vi "Caller VI_Read Icon Data From Tag.vi"(8 "Error":errorcluster, 11 "Default Body Text":T2 {"Body Text Spec"."Alignment" items=["left", "center", "right"]}) -> (0 "Error Out":errorcluster, 1 "Library Icon If Valid":picture, 2 "Who Invoked The Icon Editor? Out":T5, 3 "Data Out":T1 {"Body Text"."Body Text Spec"."Alignment" items=["left", "center", "right"]}, 4 "Valid? Out":bool, 5 "Valid Library Icon? Out":bool)   [LabVIEW 2021]
uses:
  <resource>/plugins/IconEditor/Who Invoked Icon Editor.ctl
  <resource>/plugins/IconEditor/Icon Editor Invoker Type.ctl
  TypeDefs/Cluster_BodyText.ctl
  vi.lib/LabVIEW Icon API/lv_icon/Controls/Font.ctl
  vi.lib/LabVIEW Icon API/lv_icon/Controls/Alignment.ctl
  vi.lib/LabVIEW Icon API/lv_icon/Controls/LabVIEW Icon Stored Information.ctl
  vi.lib/LabVIEW Icon API/lv_icon/Classes/Layer/Layer.lvclass
  vi.lib/LabVIEW Icon API/lv_icon/lv_icon.lvlib
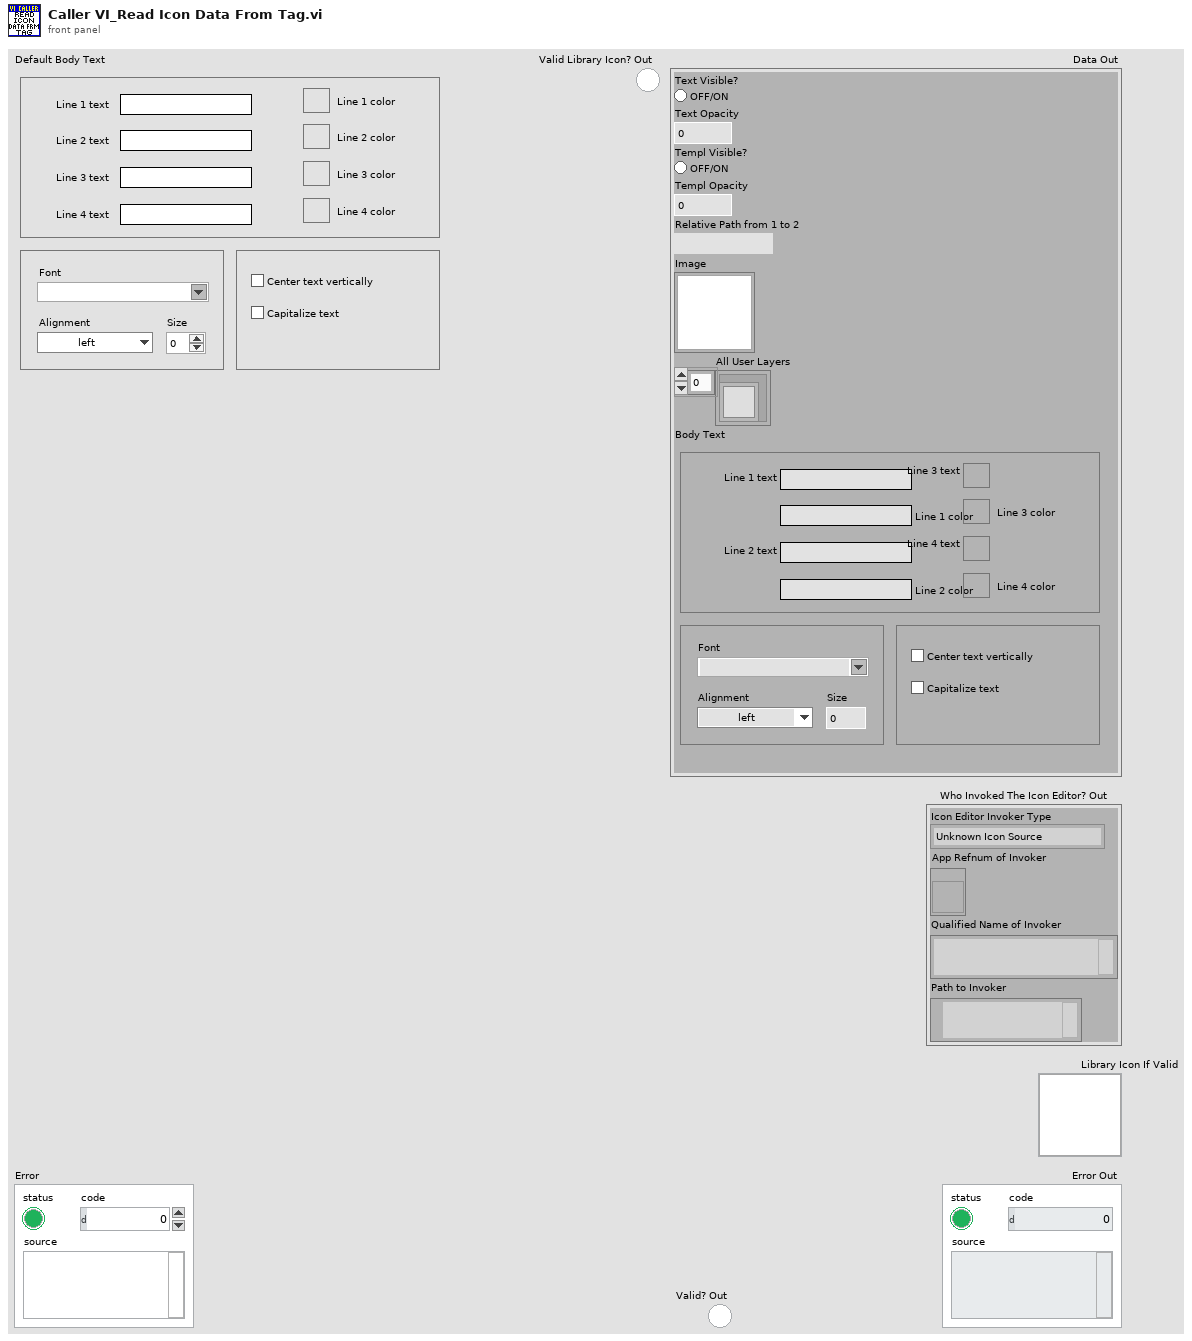
[diagram p1: front panel]
types:
  T1 = typedef "LabVIEW Icon Stored Information.ctl" = cluster{"Text Visible?":bool, "Text Opacity":u8, "Templ Visible?":bool, "Templ Opacity":u8, "Relative Path from 1 to 2":path, "Image":picture, "All User Layers":refnum<class "Layer.lvclass">[], "Body Text":T2}
  T2 = typedef "Cluster_BodyText.ctl" = cluster{"Line 1 text":string, "Line 2 text":string, "Line 3 text":string, "Line 4 text":string, "Line 1 color":u32, "Line 2 color":u32, "Line 3 color":u32, "Line 4 color":u32, "Body Text Spec":cluster{"Font":T3, "Alignment":T4, "Size":u8}, "Center text vertically":bool, "Capitalize Text":bool}
  T3 = typedef "Font.ctl" = string
  T4 = typedef "Alignment.ctl" = u16
  T5 = typedef "Who Invoked Icon Editor.ctl" = cluster{"Icon Editor Invoker Type":T6, "App Refnum of Invoker":refnum<vi>, "Qualified Name of Invoker":string, "Path to Invoker":path}
  T6 = typedef "Icon Editor Invoker Type.ctl" = enum32{"Unknown Icon Source", "VI Icon", "Library Icon (any library type)", "Palette icon", "Icon from App Method"}
  T7 = typedef "imagedata.ctl" = cluster{"image type":i32, "image depth":i32, "image":u8[], "mask":u8[], "colors":u32[], "Rectangle":cluster{"left":i16, "top":i16, "right":i16, "bottom":i16}}
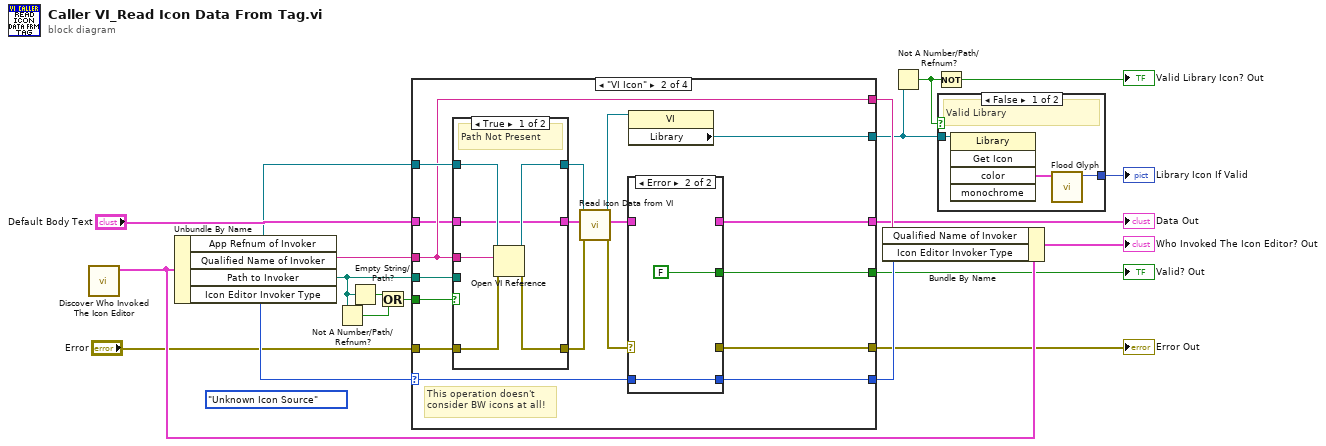
[diagram p0: block diagram]
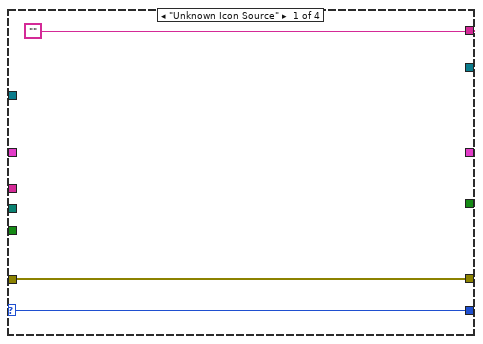
[diagram p2: hidden frame]
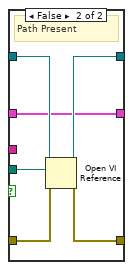
[diagram p3: hidden frame]
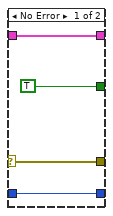
[diagram p4: hidden frame]
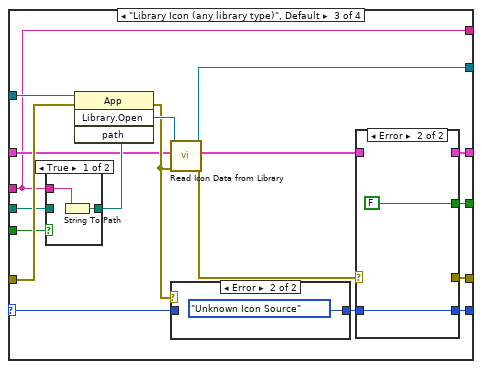
[diagram p5: hidden frame]
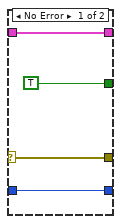
[diagram p8: hidden frame]
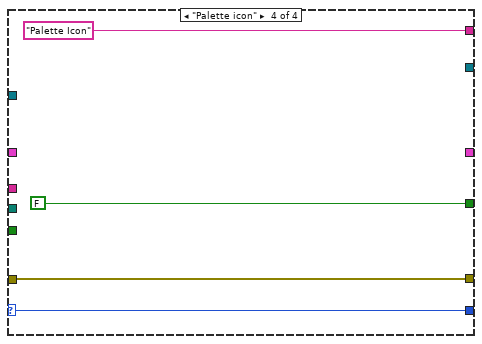
[diagram p9: hidden frame]
diagram:
  (unwired) Icon_Editor_Invoker_Type."Unknown Icon Source" ("Icon Editor Invoker Type")
  n1 = call <resource>:"Discover Who Invoked The Icon Editor.vi"() -> ("Who Invoked The Icon Editor?"=w17:T5)  [unwired: 11 out]
  n2 = Unbundle By Name(w17) -> ("App Refnum of Invoker"=w9:refnum<vi>, "Qualified Name of Invoker"=w13:string, "Path to Invoker"=w14:path, "Icon Editor Invoker Type"=w16:T6)
  n3 = Not A Number/Path/Refnum?(number/path/refnum=w14) -> (NaN/Path/Refnum?=w11:bool)
  n4 = Empty String/Path?(string/path=w14) -> (empty?=w10:bool)
  n5 = Or(x=w10, y=w11) -> (x .or. y?=w12:bool)
  n6 = case shown="\"VI Icon\"" w16 {
    selector: w16 -> [w23 w28 w65 w91]
    tunnel: [_ w39 w77 _] -> w6
    tunnel: [_ w38 w76 FALSE] -> w7
    tunnel: "Error" -> [w21 w37 w75 w89]
    tunnel: w9 -> [_ w36 w72 _]
    tunnel: [w23 w27 w63 w91] -> w19
    tunnel: w13 -> [_ w31 w66 _]
    tunnel: w14 -> [_ w33 w69 _]
    tunnel: w12 -> [_ w34 w70 _]
    tunnel: "Default Body Text" -> [_ w30 w67 _]
    tunnel: ["" w31 w66 "Palette Icon" ("String")] -> w18
    tunnel: [_ w25 w60 _] -> w1
    tunnel: [w21 w26 w62 w89] -> w2
    frame "Unknown Icon Source" {
    }
    frame "VI Icon" {
      # "This operation doesn't\nconsider BW icons at all!"
      n7 = case shown="True" w34 {
        tunnel: [w47 w53] -> w41
        tunnel: [w46 w52] -> w40
        tunnel: w37 -> [w45 w51]
        tunnel: w36 -> [w44 w50]
        tunnel: w31 -> [w43 _]
        tunnel: w33 -> [_ w49]
        tunnel: w30 -> [w42 w48]
        tunnel: [w42 w48] -> w29
        frame True {
          # "Path Not Present"
          n8 = Open VI Reference(application reference (local)=w44, vi path=w43, error in (no error)=w45) -> (vi reference=w47:refnum<vi>, error out=w46:errorcluster)  [unwired: 3 out]
        }
        frame False {
          # "Path Present"
          n9 = Open VI Reference(application reference (local)=w50, vi path=w49, error in (no error)=w51) -> (vi reference=w53:refnum<vi>, error out=w52:errorcluster)  [unwired: 3 out]
        }
      }
      n10 = call "Read Icon Data from VI.vi"("error in (no error)"=w40, "Default body text"=w29, "VI Ref in"=w41) -> ("error out"=w24:errorcluster, "Data"=w35:T1, "VI Ref out"=w32:refnum<vi>)  [unwired: 6 in]
      n11 = case shown="Error" w24 {
        selector: w24 -> [w57 _]
        tunnel: [w57 _] -> w26
        tunnel: [w55 _] -> w39
        tunnel: [TRUE FALSE] -> w38
        tunnel: w35 -> [w55 _]
        tunnel: w28 -> [w54 w58]
        tunnel: [w54 w58] -> w27
        frame No Error {
        }
        frame Error {
        }
      }
      n12 = property class="VI"(reference=w32) -> ("Library"=w25:refnum<vi>)  [unwired: 1 in, 2 out]
    }
    frame "Library Icon (any library type)", Default {
      n13 = case shown="True" w70 {
        tunnel: w69 -> [_ w80]
        tunnel: [w78 w80] -> w68
        tunnel: w66 -> [w79 _]
        frame True {
          n14 = String To Path(string=w79) -> (path=w78:path)
        }
        frame False {
        }
      }
      n15 = invoke class="App" method="Library.Open"(reference=w72, error in=w75, "path"=w68) -> (error out=w71:errorcluster, "Open Library"=w73:refnum<vi>)  [unwired: 1 in, 2 out]
      n16 = call "Read Icon Data from Library.vi"("error in (no error)"=w71, "Default body text"=w67, "Library in"=w73) -> ("error out"=w61:errorcluster, "Data"=w74:T1, "Library out"=w60:refnum<vi>)  [unwired: 6 in]
      n17 = case shown="Error" w71 {
        tunnel: [w81 Icon_Editor_Invoker_Type."Unknown Icon Source" ("Icon Editor Invoker Type")] -> w64
        tunnel: w65 -> [w81 _]
        frame No Error {
        }
        frame Error {
        }
      }
      n18 = case shown="Error" w61 {
        selector: w61 -> [w86 _]
        tunnel: [w86 _] -> w62
        tunnel: [w84 _] -> w77
        tunnel: [TRUE FALSE] -> w76
        tunnel: w74 -> [w84 _]
        tunnel: [w83 w87] -> w63
        tunnel: w64 -> [w83 w87]
        frame No Error {
        }
        frame Error {
        }
      }
    }
    frame "Palette icon" {
    }
  }
  "Valid? Out" <- w7
  "Data Out" <- w6
  "Error Out" <- w2
  n19 = Bundle By Name(cluster=w17, "Qualified Name of Invoker"=w18, "Icon Editor Invoker Type"=w19) -> (→"Who Invoked The Icon Editor? Out":T5)
  n20 = Not A Number/Path/Refnum?(number/path/refnum=w1) -> (NaN/Path/Refnum?=w3:bool)
  n21 = Not(x=w3) -> (.not. x?=→"Valid Library Icon? Out":bool)
  n22 = case shown="False" w3 {
    tunnel: [w94 _] -> w5
    tunnel: w1 -> [w93 _]
    frame False {
      # "Valid Library"
      n23 = invoke class="Library" method="Get Icon"(reference=w93) -> ("color"=w95:T7)  [unwired: 4 in, 4 out]
      n24 = call "Flood Glyph.vi"("Image Data"=w95) -> ("Pic Out"=w94:picture)  [unwired: 1 in, 9 out]
    }
    frame True {
      # "No Library"
    }
  }
  "Library Icon If Valid" <- w5
